vi "PIDF.vi"(4 "reinitialize? (F)":bool, 5 "invert? (F)":bool, 6 "PIDF gains":cluster{"Kp":dbl, "Ki":dbl, "Kd":dbl, "Kf":dbl} {"Kf" format="%.3f"; "Kd" format="%.3f"; "Ki" format="%.3f"; "Kp" format="%.3f"}, 7 "output range":cluster{"output high":dbl, "output low":dbl}={"output high"=1.0, "output low"=-1.0} {"output low" format="%.2f"; "output high" format="%.2f"}, 8 "dt (s)":dbl=0.01, 9 "i Zone":dbl=inf format="%.2f", 10 "process variable":dbl format="%.2f", 11 "setpoint":dbl format="%.2f") -> (1 "In i Zone?":bool, 2 "In Range?":bool, 3 "output":dbl format="%.2f")   [LabVIEW 2019]
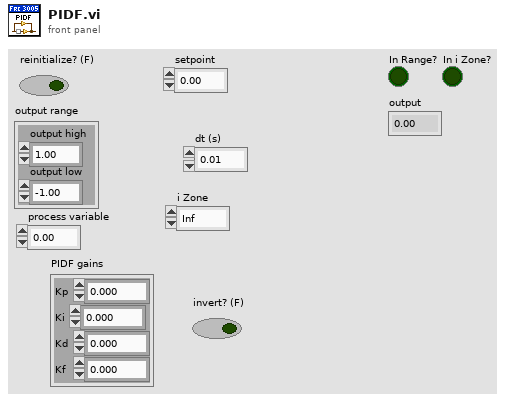
[diagram p1: front panel]
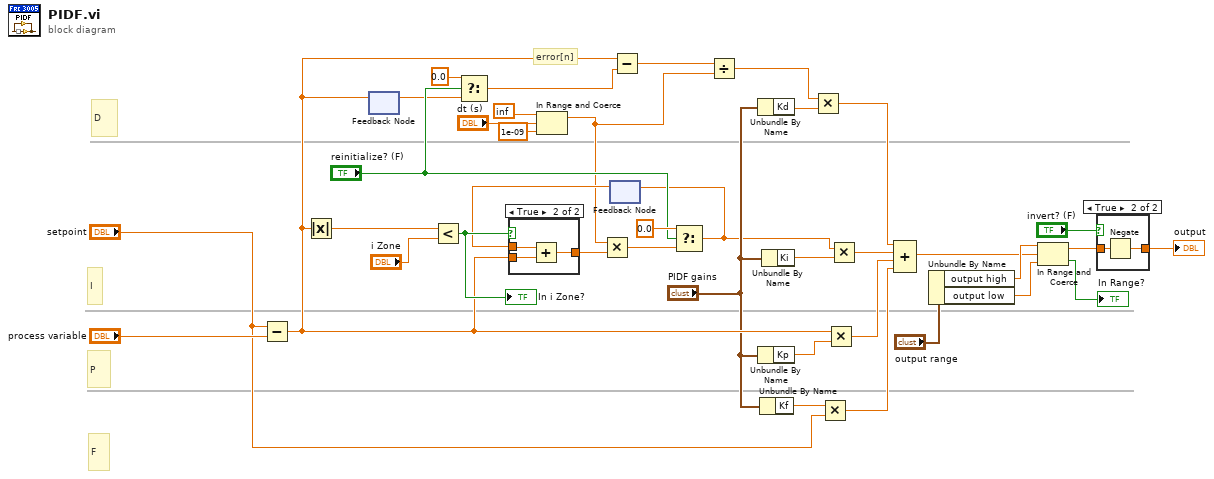
[diagram p0: block diagram]
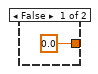
[diagram p3: hidden frame]
diagram:
  # "F"
  # "D"
  # "I"
  # "P"
  # "error[n]"
  n1 = Subtract(x="setpoint", y="process variable") -> (x-y=w30:dbl)
  n2 = Absolute Value(x=w30) -> (abs(x)=w36:dbl)
  n3 = feedback #1() -> (w28:dbl)  [unwired: 1 in]
  n4 = feedback-in #1(w30) -> ()
  n5 = Less?(x=w36, y="i Zone") -> (x < y?=w34:bool)
  "In i Zone?" <- w34
  n6 = Select(t=0.0 ("f"), s="reinitialize? (F)", f=w28) -> (s? t:f=w27:dbl)
  n7 = In Range and Coerce(upper limit=inf, x="dt (s)", lower limit=1e-09) -> (coerced(x)=w1:dbl)  [unwired: 1 out]
  n8 = feedback #2() -> (w33:dbl)  [unwired: 1 in]
  n9 = case shown="True" w34 {
    tunnel: w30 -> [_ w42]
    tunnel: [0.0 ("f") w41] -> w5
    tunnel: w33 -> [_ w40]
    frame False {
    }
    frame True {
      n10 = Add(x=w40, y=w42) -> (x+y=w41:dbl)
    }
  }
  n11 = Multiply(x=w1, y=w5) -> (x*y=w6:dbl)
  n12 = Subtract(x=w30, y=w27) -> (x-y=w8:dbl)
  n13 = Select(t=0.0 ("f"), s="reinitialize? (F)", f=w6) -> (s? t:f=w15:dbl)
  n14 = feedback-in #2(w15) -> ()
  n15 = Divide(x=w8, y=w1) -> (x/y=w7:dbl)
  n16 = Unbundle By Name("PIDF gains") -> ("Kd"=w18:dbl)
  n17 = Unbundle By Name("PIDF gains") -> ("Kp"=w37:dbl)
  n18 = Unbundle By Name("PIDF gains") -> ("Kf"=w20:dbl)
  n19 = Unbundle By Name("PIDF gains") -> ("Ki"=w16:dbl)
  n20 = Multiply(x=w7, y=w18) -> (x*y=w17:dbl)
  n21 = Multiply(x=w20, y="setpoint") -> (x*y=w19:dbl)
  n22 = Multiply(x=w30, y=w37) -> (x*y=w26:dbl)
  n23 = Multiply(x=w15, y=w16) -> (x*y=w14:dbl)
  n24 = Compound Arithmetic op=ADD(w17, w14, w26, w19) -> (w22:dbl)
  n25 = Unbundle By Name("output range") -> ("output high"=w24:dbl, "output low"=w23:dbl)
  n26 = In Range and Coerce(upper limit=w24, x=w22, lower limit=w23) -> (coerced(x)=w12:dbl, In Range?=→"In Range?":bool)
  n27 = case shown="True" "invert? (F)" {
    tunnel: w12 -> [w43 w45]
    tunnel: [w43 w44] -> w11
    frame False {
    }
    frame True {
      n28 = Negate(x=w45) -> (-x=w44:dbl)
    }
  }
  "output" <- w11
